vi "TrajectoryTest.vi"() -> ()   [LabVIEW 2017]
panel:
  in  "File Path 2":path
  out "ChosenAngle":dbl
  in  "HomeXY(pixels)":cluster{dbl, dbl}
  out "ImageOut":T1(plugin-control)
  out "Kicker XY":cluster{dbl, dbl}
  out "ChosenEnergy":dbl
  out "ChosenPathIdx":i32
  out "Puck":T2(array[cluster]) {"Position"."Y" format="%.2f"; "Position"."X" format="%.2f"}
  out "Players":T2(array[cluster]) {"Position"."Y" format="%.2f"; "Position"."X" format="%.2f"}
  out "Vertical Edges":T3(array[cluster]) {"Point2 (Real-World)"."Y" format="%.2f"; "Point2 (Real-World)"."X" format="%.2f"; "Point1 (Real-World)"."Y" format="%.2f"; "Point1 (Real-World)"."X" format="%.2f"; "Point2 (Pixels)"."Y" format="%.2f"; "Point2 (Pixels)"."X" format="%.2f"; "Point1 (Pixels)"."Y" format="%.2f"; "Point1 (Pixels)"."X" format="%.2f"}
  out "Horizontal Edges":T3(array[cluster]) {"Point2 (Real-World)"."Y" format="%.2f"; "Point2 (Real-World)"."X" format="%.2f"; "Point1 (Real-World)"."Y" format="%.2f"; "Point1 (Real-World)"."X" format="%.2f"; "Point2 (Pixels)"."Y" format="%.2f"; "Point2 (Pixels)"."X" format="%.2f"; "Point1 (Pixels)"."Y" format="%.2f"; "Point1 (Pixels)"."X" format="%.2f"}
  out "Image Out":T1(plugin-control)
  out "error out":errorcluster
  in  "File Path":path
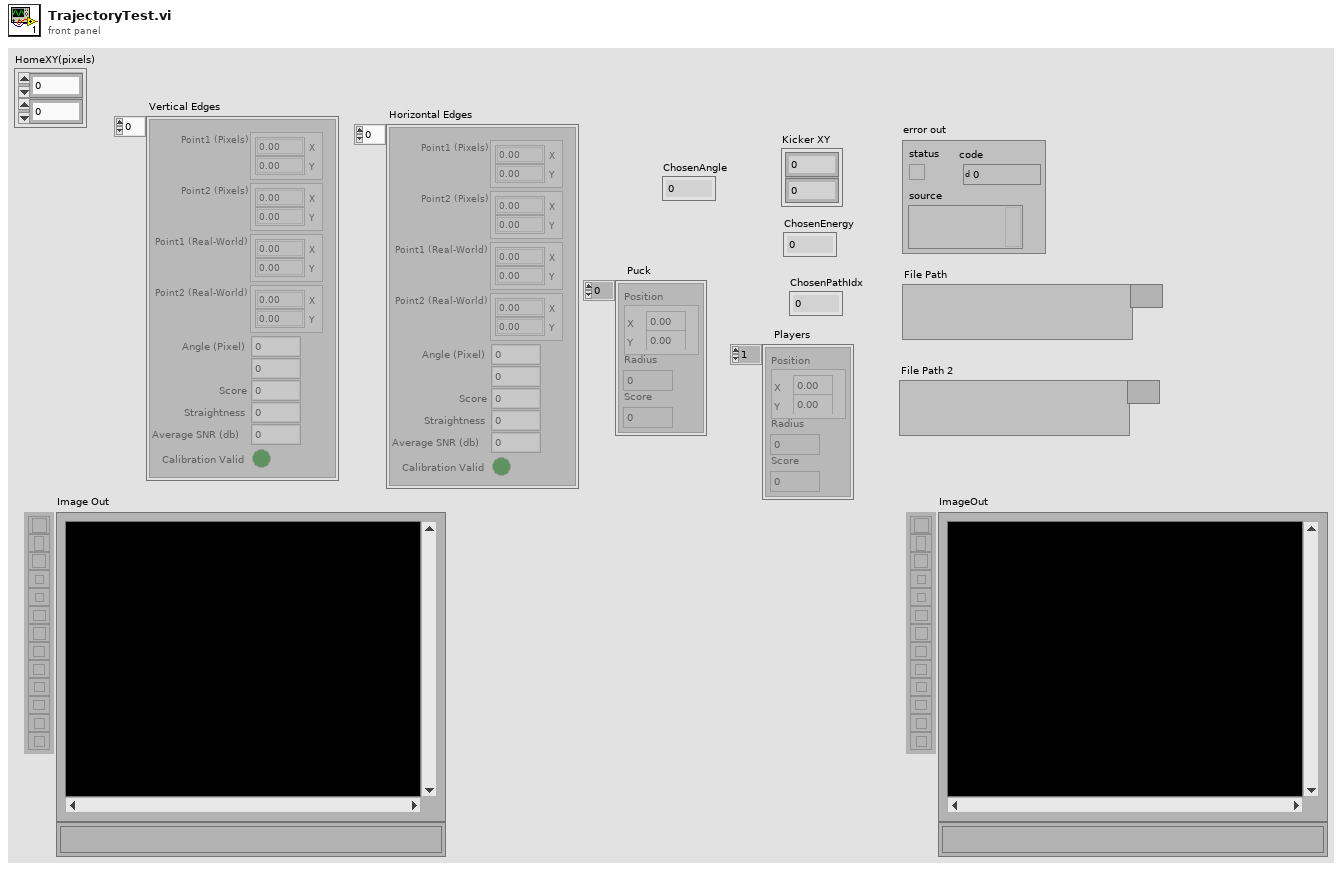
[diagram p1: front panel]
types:
  T1 = typedef "IMAQ Image.ctl" = refnum<image>
  T2 = cluster{"Position":cluster{"X":sgl, "Y":sgl}, "Radius":dbl, "Score":dbl}[]
  T3 = cluster{"Point1 (Pixels)":cluster{"X":sgl, "Y":sgl}, "Point2 (Pixels)":cluster{"X":sgl, "Y":sgl}, "Point1 (Real-World)":cluster{"X":sgl, "Y":sgl}, "Point2 (Real-World)":cluster{"X":sgl, "Y":sgl}, "Angle (Pixel)":dbl, "Angle (Real-World)":dbl, "Score":dbl, "Straightness":dbl, "Average SNR (db)":dbl, "Calibration Valid":bool}[]
  T4 = typedef "IMAQ Coordinate System" = cluster{"Reference System":cluster{"Origin":cluster{"X":sgl, "Y":sgl}, "Angle (deg)":sgl, "Axis Reference":u32}, "Measurement System":cluster{"Origin":cluster{"X":sgl, "Y":sgl}, "Angle (deg)":sgl, "Axis Reference":u32}}
  T5 = cluster{"Ptwx":dbl[], "Ptwy":dbl[], "Ptfx":dbl[], "Ptfy":dbl[], "DorR":i32[]}
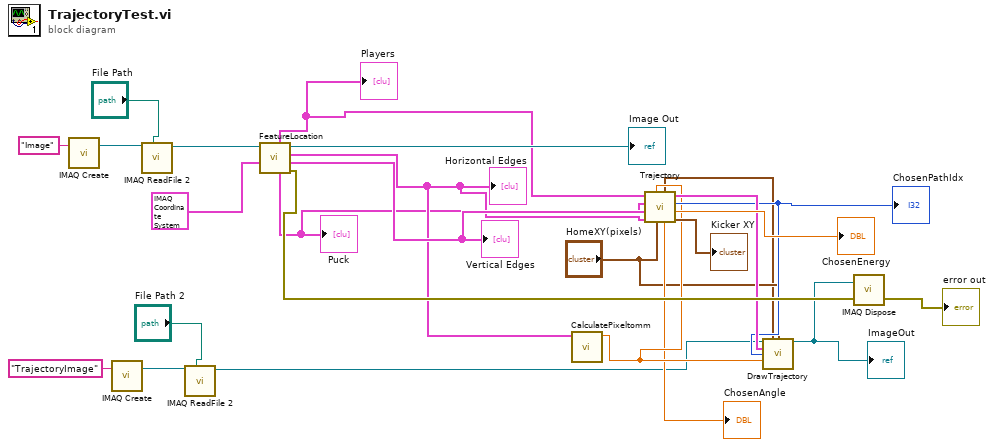
[diagram p0: block diagram]
diagram:
  n1 = call "IMAQ Create"("Image Name"="Image") -> ("New Image"=w23:T1)  [unwired: 4 in, 1 out]
  n2 = call "IMAQ Create"("Image Name"="TrajectoryImage") -> ("New Image"=w7:T1)  [unwired: 4 in, 1 out]
  n3 = call "IMAQ ReadFile 2"("File Path"="File Path", "Image"=w23) -> ("Image Out"=w10:T1)  [unwired: 5 in, 4 out]
  n4 = call "IMAQ ReadFile 2"("File Path"="File Path 2", "Image"=w7) -> ("Image Out"=w5:T1)  [unwired: 5 in, 4 out]
  n5 = call "FeatureLocation.vi"("Coordinate System"=T4 {"Reference System"={"Origin"={"X"=0.0, "Y"=0.0}, "Angle (deg)"=0.0, "Axis Reference"=0}, "Measurement System"={"Origin"={"X"=0.0, "Y"=0.0}, "Angle (deg)"=0.0, "Axis Reference"=0}}, "Image"=w10) -> ("error out"=w22:errorcluster, "Vertical Edges"=w21:T3, "Horizontal Edges"=w18:T3, "Image 2"=→"Image Out":T1, "Puck"=w2:T2, "Players"=w3:T2)  [unwired: 4 in]
  "Horizontal Edges" <- w18
  "Vertical Edges" <- w21
  "Players" <- w3
  "Puck" <- w2
  n6 = call "CalculatePixeltomm.vi"("Horizontal Edges"=w18) -> ("Pixel/mm"=w12:dbl)  [unwired: 10 in]
  n7 = call "Trajectory.vi"("HomeXY(pixels)"="HomeXY(pixels)", "PixelmmRatio"=w12, "Horizontal Edges"=w18, "Vertical Edges"=w21, "Puck"=w2, "Players"=w3) -> ("Kicker XY"=→"Kicker XY":cluster{dbl, dbl}, "ChosenEnergy"=→"ChosenEnergy":dbl, "ChosenPathIdx"=w15:i32, "TrajectoryArray"=w17:T5, "Angle"=→"ChosenAngle":dbl, "PuckCentre"=w1:cluster{"PuckX":sgl, "PuckY":sgl})
  "ChosenPathIdx" <- w15
  n8 = call "DrawTrajectory.vi"("Image"=w5, "PuckCentre"=w1, "HomePoint(pixels)"="HomeXY(pixels)", "TrajectoryArray"=w17, "ChosenPath"=w15, "Pixel/mm"=w12) -> ("ImageOut"=w14:T1)  [unwired: 8 in, 1 out]
  "ImageOut" <- w14
  n9 = call "IMAQ Dispose"("Image"=w14, "error in (no error)"=w22) -> ("error out"=→"error out":errorcluster)  [unwired: 4 in]
